vi "Tab Page Color.vi"() -> ()   [LabVIEW 2022 SP3]
panel:
  in  "Tab Control":enum32{"Page 1", "Page 2"}(tab)
  in  "Thermometer":dbl(slide) scale=0.0..100.0
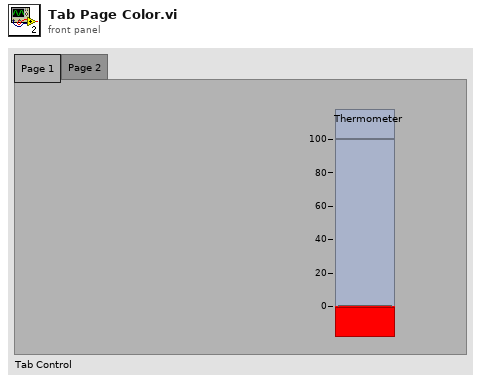
[diagram p1: front panel]
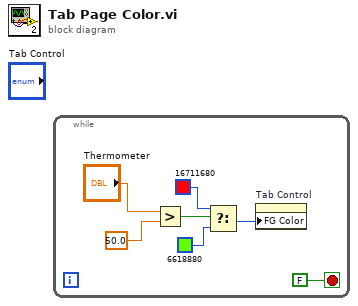
[diagram p0: block diagram]
diagram:
  n1 = while {
    stop <- FALSE stop-if-true
    n2 = Greater?(x="Thermometer", y=50.0) -> (0:w4:bool)
    n3 = Select(t=u32 16711680, s=w4, f=u32 6618880) -> (s? t:f=w1:u32)
    n4 = property on="Tab Control" class="TabCtl (strict)"("FG Color"=w1) -> ()  [unwired: 2 in, 2 out]
  }
